vi "packing.vi"(8 "error in (no error)":errorcluster, 11 "Burger in":refnum<class "Burger.lvclass">) -> (0 "error out":errorcluster, 2 "Packing.lvclass":refnum<class "Packing.lvclass">, 3 "Burger out":refnum<class "Burger.lvclass">)   [LabVIEW 2018, in "Burger.lvclass"]
uses:
  Burger.lvclass
  Packing Class/Packing.lvclass
  Wrapper Class/Wrapper.lvclass
  C:/Users/fflores/Documents/LabVIEW-Open-Projects/LabIVEW OOP Design Patterns/Builder Pattern/Packing Class/Packing.lvclass
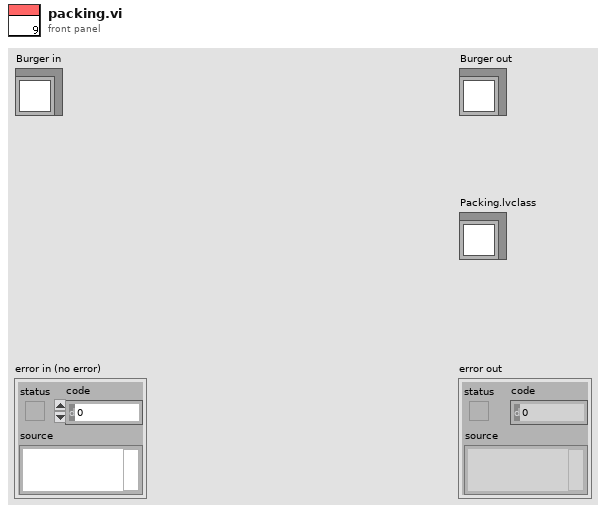
[diagram p1: front panel]
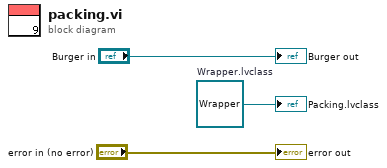
[diagram p0: block diagram]
diagram:
  w1 = refnum<class "Wrapper.lvclass"> refnum  # Wrapper.lvclass
  "error out" <- "error in (no error)"
  "Burger out" <- "Burger in"
  "Packing.lvclass" <- w1
